vi "SUMMER SUNDAY FINAL[test].vi"() -> ()   [LabVIEW 2009]
uses:
  <vilib>/ULx/Create Channel.llb/ULx Create Channel (AI-Voltage-Basic).vi
  <vilib>/ULx/Create Channel.llb/ULx Create Channel (DO-Digital Output).vi
  <vilib>/ULx/Create Channel.llb/ULx Create Channel (DI-Digital Input).vi
  <vilib>/ULx/Write.llb/ULx Write (Digital Bool 1Line 1Point).vi
  <vilib>/ULx/Read.llb/ULx Read (Analog DBL 1Chan 1Samp).vi
  <vilib>/ULx/Read.llb/ULx Read (Digital 1D U8 NChan 1Samp).vi
panel:
  in  "Reset":bool
  out "POWER":bool
  out "ENERGY LEVEL":dbl(knob) scale=0.0..15.0
  out "READY 2":bool
  out "DUMP":bool
  out "POWER":bool
  out "?":bool
  out "?":bool
  out "?":bool
  out "?":bool
  out "?":bool
  out "?":bool
  out "?":bool
  out "?":bool
  out "?":bool
  out "?":bool
  out "OPEN":bool
  out "CLOSED":bool
  out "READY":bool
  out "FAULT":bool
  out "MAGNET FORCE":dbl(slide) scale=0.0..10.0
  out "READY":bool
  out "TEMPERATURE":dbl(slide) scale=0.0..100.0
  in  "stop":bool
  out "?":bool
  out "?":bool
  out "?":bool
  out "?":bool
  out "FAULT":bool
  out "POWER":bool
  out "FLOW IN GPM":dbl(knob) scale=0.0..15.0
  # "USERS LAB AREA"
  # "BEAM STATUS"
  # "ROOM"
  # "XRAY"
  # "PUMP STATION"
  # "MAGNET STATUS"
  # "ORBIT"
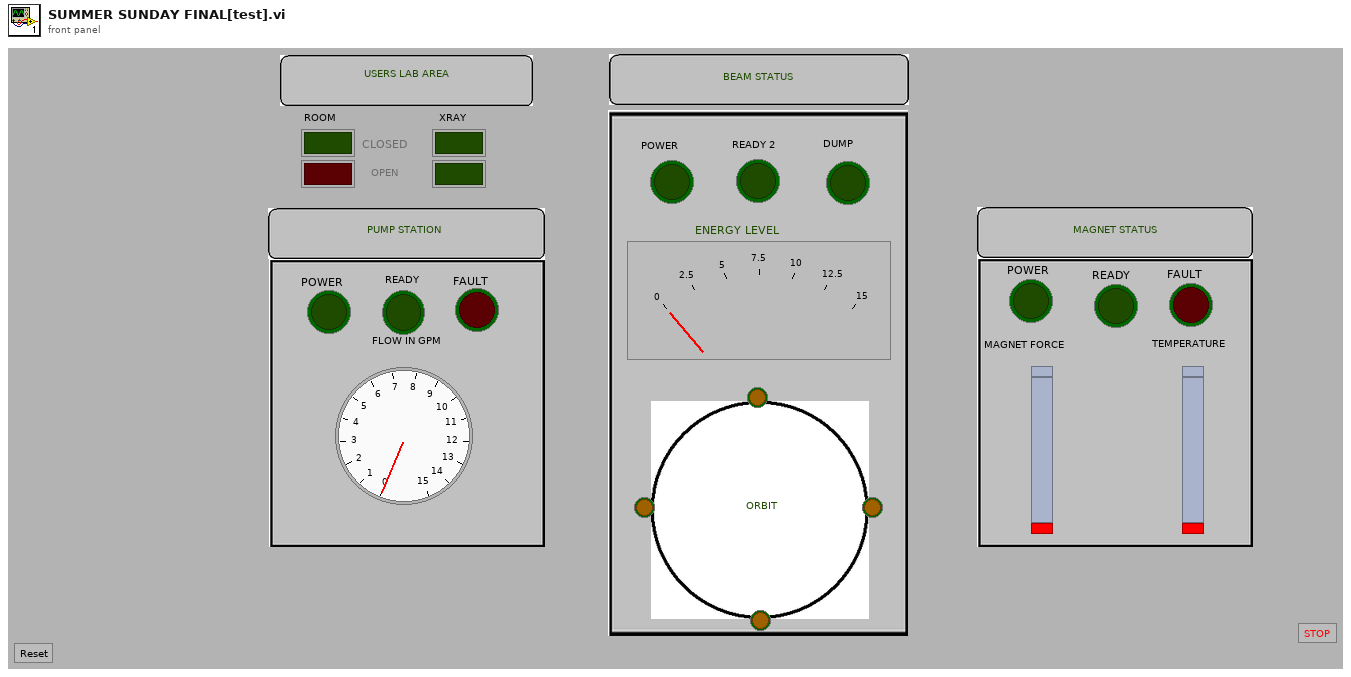
[diagram p1: front panel]
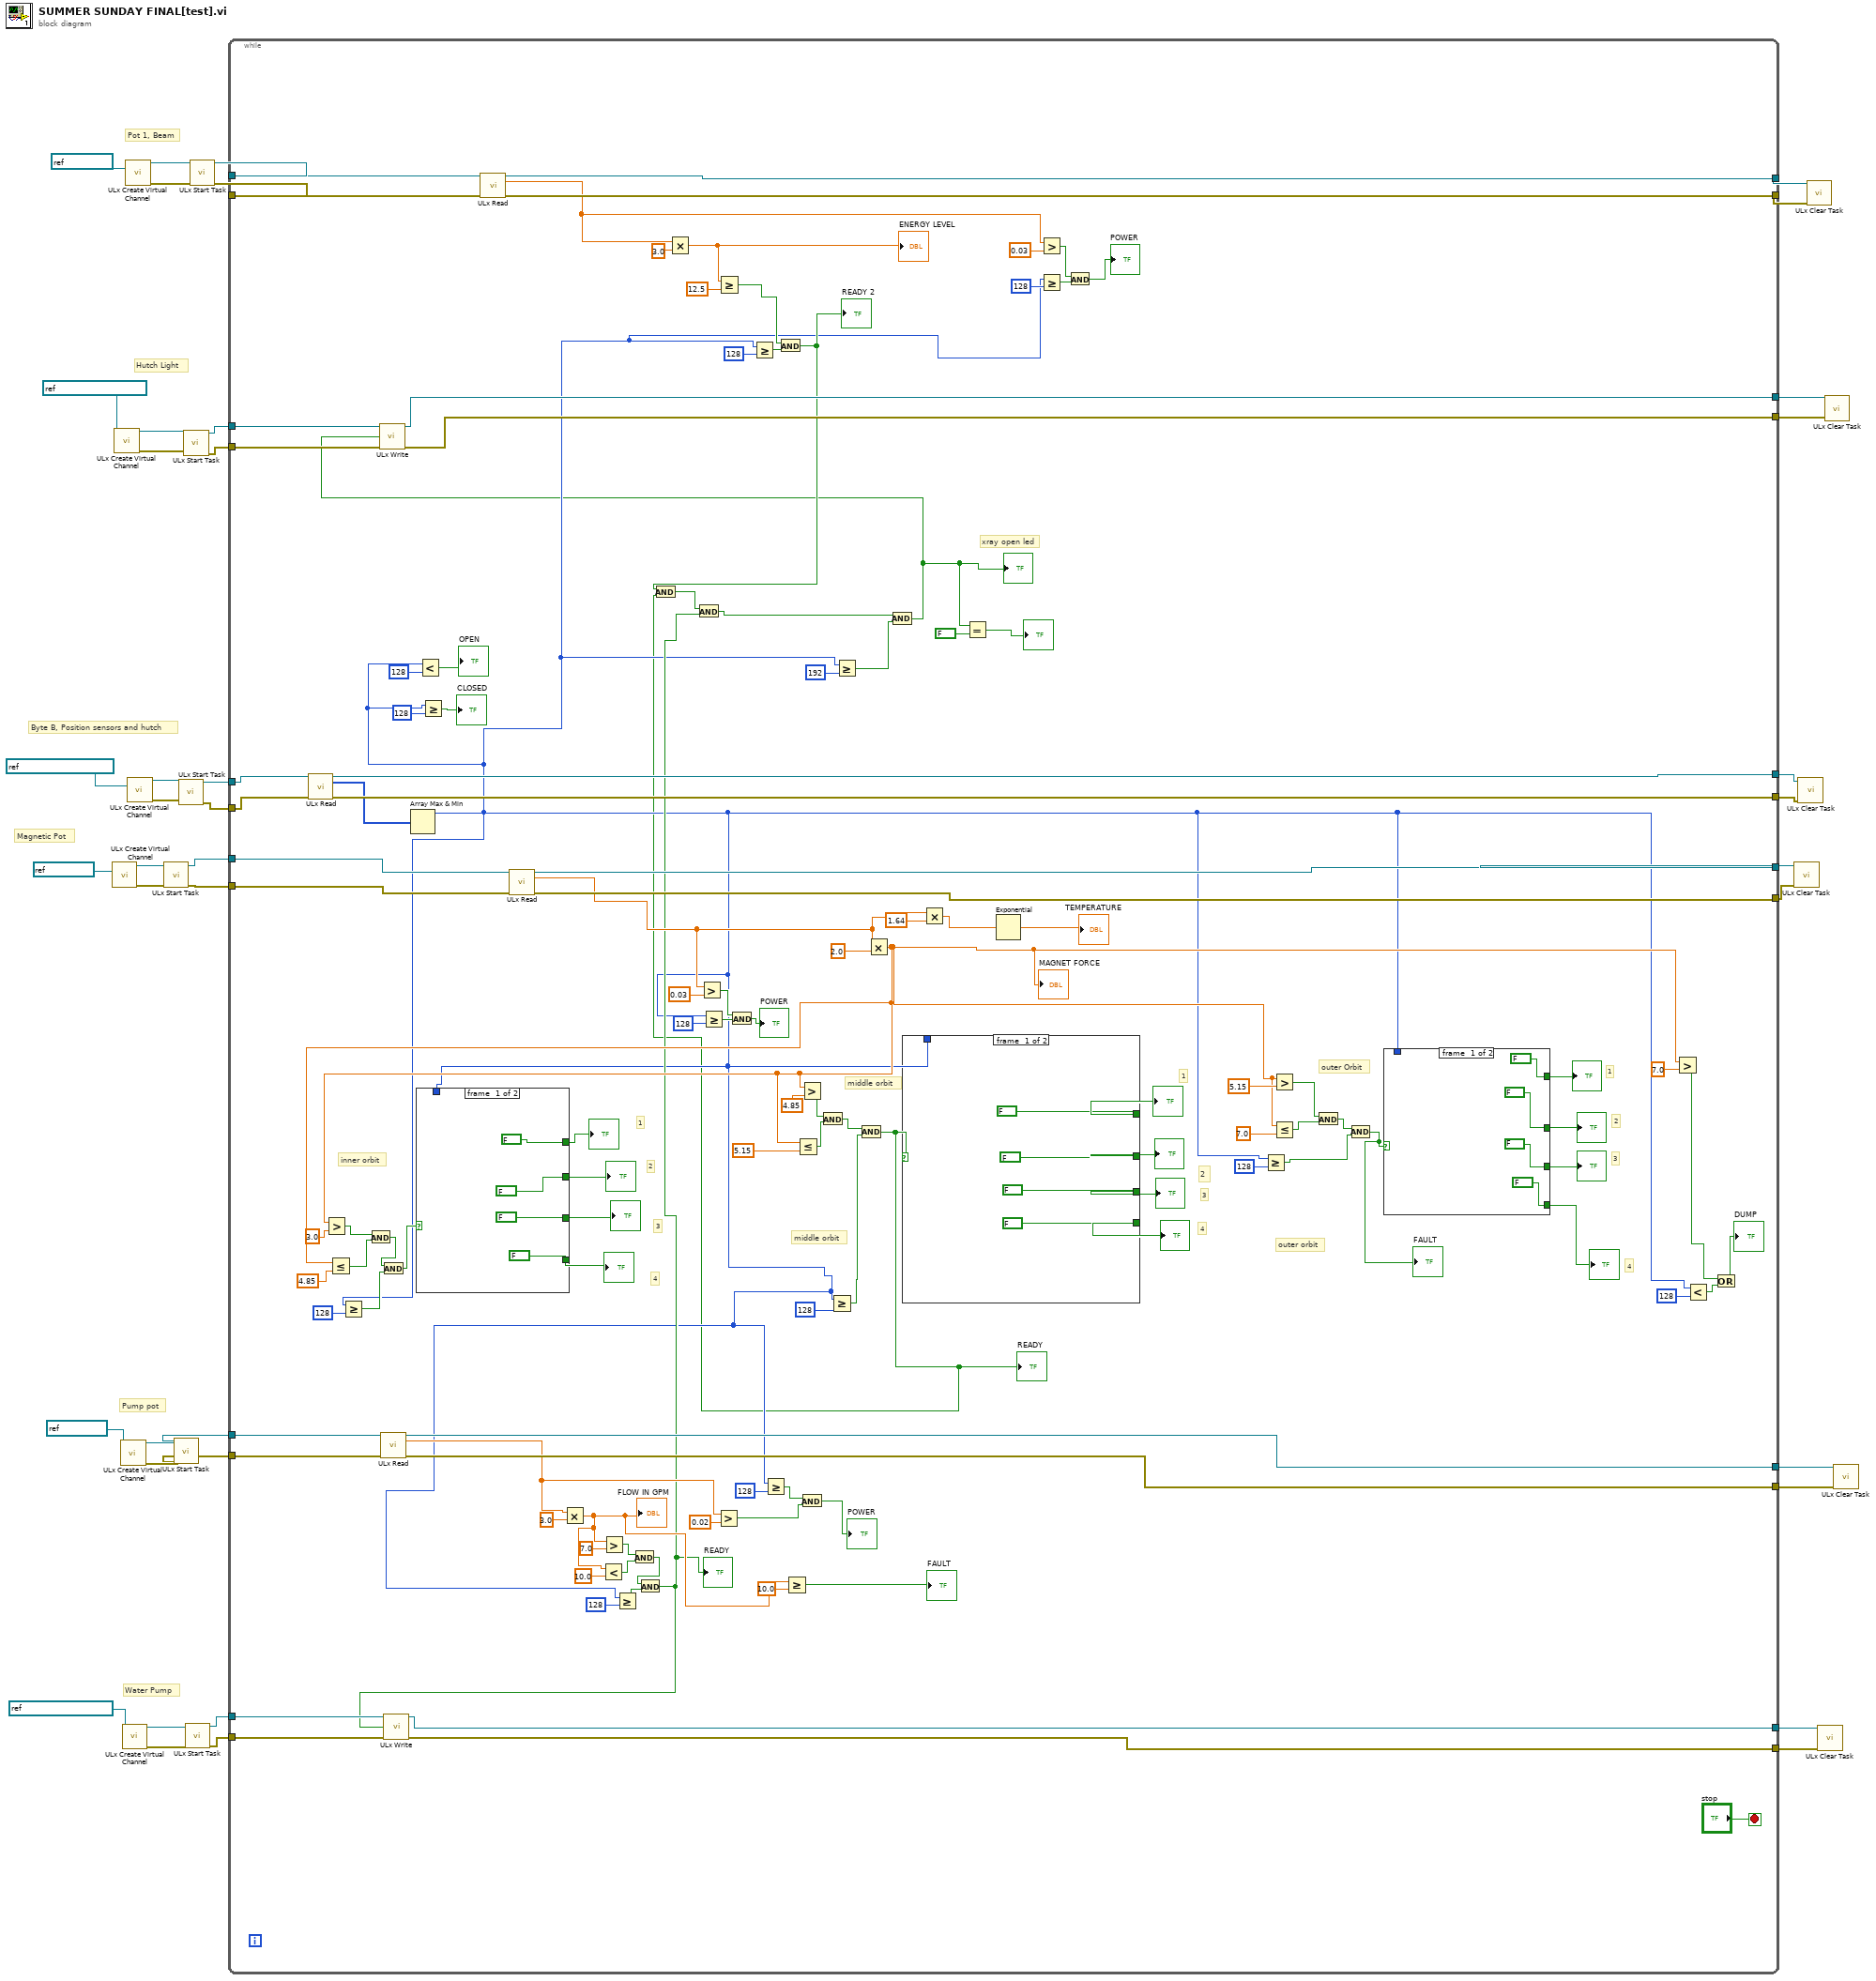
[diagram p0: block diagram]
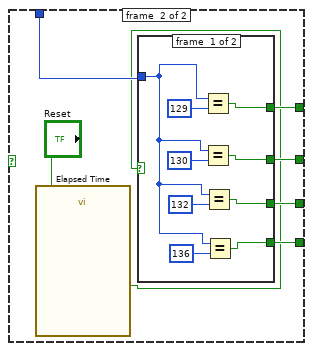
[diagram p2: hidden frame]
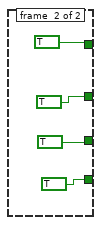
[diagram p3: hidden frame]
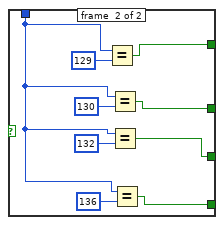
[diagram p4: hidden frame]
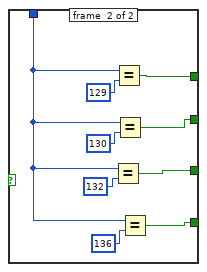
[diagram p5: hidden frame]
diagram:
  # "Water Pump"
  # "Pump pot"
  # "Hutch Light"
  # "Byte B, Position sensors and hutch"
  # "Magnetic Pot"
  # "Pot 1, Beam"
  n1 = call-poly <vilib>:"ULx Create Virtual Channel.vi"("physical channels"=refnum<k21> "Dev0/Ai1") -> ("task out"=w36:refnum<k24>, "error out"=w35:errorcluster)  [unwired: 13 in]
  n2 = call-poly <vilib>:"ULx Create Virtual Channel.vi"("lines"=refnum<k21> "Dev0/1stPortA/Do0") -> ("task out"=w21:refnum<k24>, "error out"=w20:errorcluster)  [unwired: 13 in]
  n3 = call-poly <vilib>:"ULx Create Virtual Channel.vi"("physical channels"=refnum<k21> "Dev0/Ai2") -> ("task out"=w28:refnum<k24>, "error out"=w27:errorcluster)  [unwired: 13 in]
  n4 = call-poly <vilib>:"ULx Create Virtual Channel.vi"("lines"=refnum<k21> "Dev0/1stPortA/Do1") -> ("task out"=w7:refnum<k24>, "error out"=w6:errorcluster)  [unwired: 13 in]
  n5 = call-poly <vilib>:"ULx Create Virtual Channel.vi"("physical channels"=refnum<k21> "Dev0/Ai0") -> ("task out"=w42:refnum<k24>, "error out"=w41:errorcluster)  [unwired: 13 in]
  n6 = call-poly <vilib>:"ULx Create Virtual Channel.vi"("lines"=refnum<k21> "Dev0/1stPortB/Di0:7") -> ("task out"=w14:refnum<k24>, "error out"=w13:errorcluster)  [unwired: 13 in]
  n7 = call <vilib>:"ULx Start Task.vi"("task in"=w36, "error in"=w35) -> ("task out"=w34:refnum<k24>, "error out"=w33:errorcluster)  [unwired: 12 in]
  n8 = call <vilib>:"ULx Start Task.vi"("task in"=w28, "error in"=w27) -> ("task out"=w26:refnum<k24>, "error out"=w25:errorcluster)  [unwired: 12 in]
  n9 = call <vilib>:"ULx Start Task.vi"("task in"=w14, "error in"=w13) -> ("task out"=w12:refnum<k24>, "error out"=w11:errorcluster)  [unwired: 12 in]
  n10 = call <vilib>:"ULx Start Task.vi"("task in"=w21, "error in"=w20) -> ("task out"=w18:refnum<k24>, "error out"=w17:errorcluster)  [unwired: 12 in]
  n11 = call <vilib>:"ULx Start Task.vi"("task in"=w7, "error in"=w6) -> ("task out"=w5:refnum<k24>, "error out"=w4:errorcluster)  [unwired: 12 in]
  n12 = call <vilib>:"ULx Start Task.vi"("task in"=w42, "error in"=w41) -> ("task out"=w40:refnum<k24>, "error out"=w39:errorcluster)  [unwired: 12 in]
  n13 = while {
    tunnel: w40 -> [w162]
    tunnel: w39 -> [w161]
    tunnel: [w160] -> w38
    tunnel: [w159] -> w37
    tunnel: w34 -> [w157]
    tunnel: w33 -> [w156]
    tunnel: [w155] -> w32
    tunnel: [w154] -> w31
    tunnel: w26 -> [w116]
    tunnel: w25 -> [w115]
    tunnel: [w114] -> w23
    tunnel: [w113] -> w22
    tunnel: w18 -> [w91]
    tunnel: w17 -> [w90]
    tunnel: [w89] -> w16
    tunnel: [w88] -> w15
    tunnel: w12 -> [w87]
    tunnel: w11 -> [w86]
    tunnel: [w85] -> w9
    tunnel: [w84] -> w8
    tunnel: w5 -> [w60]
    tunnel: w4 -> [w59]
    tunnel: [w58] -> w3
    tunnel: [w57] -> w2
    stop <- "stop" stop-if-true
    # "xray open led"
    # "outer Orbit"
    # "middle orbit"
    # "4"
    # "3"
    # "2"
    # "1"
    # "1"
    # "2"
    # "3"
    # "4"
    # "4"
    # "3"
    # "2"
    # "1"
    # "outer orbit"
    # "inner orbit"
    # "middle orbit"
    n14 = call-poly <vilib>:"ULx Read.vi"("task in"=w87, "error in"=w86) -> ("task out"=w85:refnum<k24>, "data"=w83:u8[], "error out"=w84:errorcluster)  [unwired: 11 in]
    n15 = call-poly <vilib>:"ULx Read.vi"("task in"=w116, "error in"=w115) -> ("task out"=w114:refnum<k24>, "data"=w109:dbl, "error out"=w113:errorcluster)  [unwired: 11 in]
    n16 = Array Max & Min(array=w83) -> (max value=w48:u8)  [unwired: 3 out]
    n17 = Greater Or Equal?(x=w48, y=i16 128) -> (x >= y?=w141:bool)
    n18 = Less?(x=w48, y=u8 128) -> (x < y?=→"OPEN":bool)
    n19 = Greater Or Equal?(x=w48, y=u8 128) -> (x >= y?=→"CLOSED":bool)
    n20 = call-poly <vilib>:"ULx Read.vi"("task in"=w162, "error in"=w161) -> ("task out"=w160:refnum<k24>, "data"=w50:dbl, "error out"=w159:errorcluster)  [unwired: 11 in]
    n21 = call-poly <vilib>:"ULx Read.vi"("task in"=w157, "error in"=w156) -> ("task out"=w155:refnum<k24>, "data"=w95:dbl, "error out"=w154:errorcluster)  [unwired: 11 in]
    n22 = Multiply(x=w109, y=3.0) -> (x*y=w101:dbl)
    "FLOW IN GPM" <- w101
    n23 = Less?(x=w101, y=10.0) -> (x < y?=w99:bool)
    n24 = Greater?(x=w101, y=7.0) -> (0:w100:bool)
    n25 = Greater Or Equal?(x=w48, y=u8 128) -> (x >= y?=w74:bool)
    n26 = And(x=w100, y=w99) -> (x .and. y?=w72:bool)
    n27 = And(x=w72, y=w74) -> (x .and. y?=w52:bool)
    "READY" <- w52
    n28 = call-poly <vilib>:"ULx Write.vi"("task in"=w60, "data"=w52, "error in"=w59) -> ("task out"=w58:refnum<k24>, "error out"=w57:errorcluster)  [unwired: 10 in, 1 out]
    n29 = Multiply(x=w50, y=3.0) -> (x*y=w106:dbl)
    "ENERGY LEVEL" <- w106
    n30 = Greater?(x=w95, y=0.03) -> (0:w77:bool)
    n31 = Greater Or Equal?(x=w48, y=u8 128) -> (x >= y?=w76:bool)
    n32 = Greater?(x=w109, y=0.02) -> (0:w69:bool)
    n33 = Greater Or Equal?(x=w106, y=12.5) -> (x >= y?=w49:bool)
    n34 = And(x=w77, y=w76) -> (x .and. y?=→"POWER":bool)
    n35 = Greater Or Equal?(x=w48, y=u8 128) -> (x >= y?=w66:bool)
    n36 = Greater Or Equal?(x=w48, y=u8 128) -> (x >= y?=w70:bool)
    n37 = And(x=w49, y=w66) -> (x .and. y?=w64:bool)
    "READY 2" <- w64
    n38 = Greater Or Equal?(x=w101, y=10.0) -> (x >= y?=→"FAULT":bool)
    n39 = And(x=w70, y=w69) -> (x .and. y?=→"POWER":bool)
    n40 = Greater Or Equal?(x=w48, y=i16 128) -> (x >= y?=w82:bool)
    n41 = Greater Or Equal?(x=w48, y=u8 192) -> (x >= y?=w78:bool)
    n42 = Multiply(x=w95, y=2.0) -> (x*y=w134:dbl)
    "MAGNET FORCE" <- w134
    n43 = Greater?(x=w134, y=3.0) -> (0:w150:bool)
    n44 = Less Or Equal?(x=w134, y=4.85) -> (x <= y?=w151:bool)
    n45 = And(x=w150, y=w151) -> (x .and. y?=w143:bool)
    n46 = And(x=w143, y=w141) -> (x .and. y?=w142:bool)
    n47 = case shown="True" w142 {
      tunnel: [FALSE w208] -> w119
      tunnel: [FALSE w207] -> w120
      tunnel: [FALSE w206] -> w117
      tunnel: [FALSE w205] -> w118
      tunnel: w48 -> [_ w213]
      frame #0 {
      }
      frame #1 {
        n48 = Equal?(x=w213, y=i16 132) -> (x = y?=w206:bool)
        n49 = Equal?(x=w213, y=i16 129) -> (x = y?=w208:bool)
        n50 = Equal?(x=w213, y=i16 130) -> (x = y?=w207:bool)
        n51 = Equal?(x=w213, y=i16 136) -> (x = y?=w205:bool)
      }
    }
    "?" <- w120
    "?" <- w117
    "?" <- w118
    "?" <- w119
    n52 = Less Or Equal?(x=w134, y=5.15) -> (x <= y?=w147:bool)
    n53 = Greater?(x=w134, y=4.85) -> (0:w148:bool)
    n54 = And(x=w148, y=w147) -> (x .and. y?=w140:bool)
    n55 = And(x=w140, y=w82) -> (x .and. y?=w43:bool)
    "READY" <- w43
    n56 = And(x=w64, y=w43) -> (x .and. y?=w80:bool)
    n57 = And(x=w80, y=w52) -> (x .and. y?=w79:bool)
    n58 = And(x=w79, y=w78) -> (x .and. y?=w46:bool)
    "?" <- w46
    n59 = call-poly <vilib>:"ULx Write.vi"("task in"=w91, "data"=w46, "error in"=w90) -> ("task out"=w89:refnum<k24>, "error out"=w88:errorcluster)  [unwired: 10 in, 1 out]
    n60 = case shown="True" w43 {
      tunnel: [FALSE w174] -> w129
      tunnel: [FALSE w173] -> w128
      tunnel: [FALSE w172] -> w127
      tunnel: [FALSE w171] -> w126
      tunnel: w48 -> [_ w170]
      frame #0 {
      }
      frame #1 {
        n61 = call "Elapsed Time"("Reset"="Reset") -> ("Time has Elapsed"=w169:bool)  [unwired: 11 in, 7 out]
        n62 = case shown="False" w169 {
          tunnel: [w178 TRUE] -> w174
          tunnel: [w177 TRUE] -> w173
          tunnel: [w176 TRUE] -> w172
          tunnel: [w175 TRUE] -> w171
          tunnel: w170 -> [w179 _]
          frame #0 {
            n63 = Equal?(x=w179, y=i16 129) -> (x = y?=w178:bool)
            n64 = Equal?(x=w179, y=i16 130) -> (x = y?=w177:bool)
            n65 = Equal?(x=w179, y=i16 132) -> (x = y?=w176:bool)
            n66 = Equal?(x=w179, y=i16 136) -> (x = y?=w175:bool)
          }
          frame #1 {
          }
        }
      }
    }
    "?" <- w129
    "?" <- w128
    "?" <- w127
    "?" <- w126
    n67 = Multiply(x=w95, y=1.64) -> (x*y=w93:dbl)
    n68 = Equal?(x=w46, y=FALSE) -> (x = y?=→"?":bool)
    n69 = Exponential(1:w93) -> (0:→"TEMPERATURE":dbl)
    n70 = Greater?(x=w50, y=0.03) -> (0:w62:bool)
    n71 = Greater Or Equal?(x=w48, y=u8 128) -> (x >= y?=w67:bool)
    n72 = And(x=w62, y=w67) -> (x .and. y?=→"POWER":bool)
    n73 = Greater Or Equal?(x=w48, y=i16 128) -> (x >= y?=w124:bool)
    n74 = Greater?(x=w134, y=5.15) -> (0:w145:bool)
    n75 = Less Or Equal?(x=w134, y=7.0) -> (x <= y?=w144:bool)
    n76 = And(x=w145, y=w144) -> (x .and. y?=w133:bool)
    n77 = And(x=w133, y=w124) -> (x .and. y?=w96:bool)
    "FAULT" <- w96
    n78 = case shown="True" w96 {
      tunnel: [FALSE w192] -> w138
      tunnel: [FALSE w193] -> w137
      tunnel: [FALSE w194] -> w136
      tunnel: [FALSE w195] -> w135
      tunnel: w48 -> [_ w200]
      frame #0 {
      }
      frame #1 {
        n79 = Equal?(x=w200, y=i16 129) -> (x = y?=w195:bool)
        n80 = Equal?(x=w200, y=i16 130) -> (x = y?=w194:bool)
        n81 = Equal?(x=w200, y=i16 132) -> (x = y?=w193:bool)
        n82 = Equal?(x=w200, y=i16 136) -> (x = y?=w192:bool)
      }
    }
    "?" <- w135
    "?" <- w136
    "?" <- w137
    "?" <- w138
    n83 = Greater?(x=w134, y=7.0) -> (0:w97:bool)
    n84 = Less?(x=w48, y=i16 128) -> (x < y?=w121:bool)
    n85 = Or(x=w97, y=w121) -> (x .or. y?=→"DUMP":bool)
  }
  n86 = call <vilib>:"ULx Clear Task.vi"("task in"=w32, "error in"=w31) -> ()  [unwired: 13 in, 1 out]
  n87 = call <vilib>:"ULx Clear Task.vi"("task in"=w9, "error in"=w8) -> ()  [unwired: 13 in, 1 out]
  n88 = call <vilib>:"ULx Clear Task.vi"("task in"=w38, "error in"=w37) -> ()  [unwired: 13 in, 1 out]
  n89 = call <vilib>:"ULx Clear Task.vi"("task in"=w3, "error in"=w2) -> ()  [unwired: 13 in, 1 out]
  n90 = call <vilib>:"ULx Clear Task.vi"("task in"=w16, "error in"=w15) -> ()  [unwired: 13 in, 1 out]
  n91 = call <vilib>:"ULx Clear Task.vi"("task in"=w23, "error in"=w22) -> ()  [unwired: 13 in, 1 out]
